vi "NumericOps2.vi"() -> ()   [LabVIEW 2019]
panel:
  out "sqrt(x)":dbl
  out "x-1":dbl
  out "x+1":dbl
  in  "Num3":dbl
  out "floor(x/y)":dbl
  out "x-y*floor(x/y)":dbl
  in  "Num2":dbl
  in  "Num1":dbl
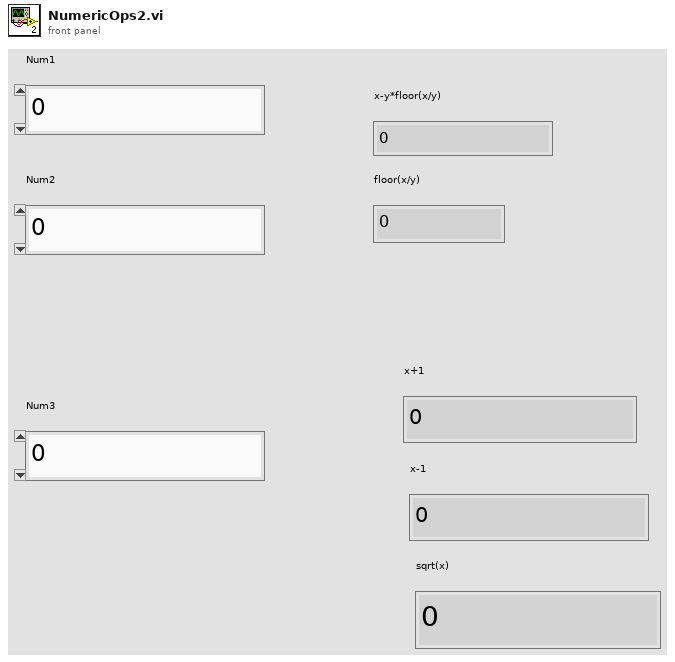
[diagram p1: front panel]
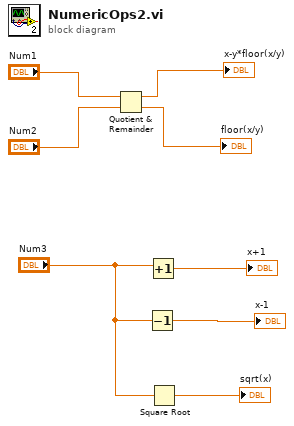
[diagram p0: block diagram]
diagram:
  n1 = Quotient & Remainder(x="Num1", y="Num2") -> (x-y*floor(x/y)=→"x-y*floor(x/y)":dbl, floor(x/y)=→"floor(x/y)":dbl)
  n2 = Decrement(x="Num3") -> (x-1=→"x-1":dbl)
  n3 = Increment(x="Num3") -> (x+1=→"x+1":dbl)
  n4 = Square Root(x="Num3") -> (sqrt(x)=→"sqrt(x)":dbl)
